vi "B_GetProperty.vi"(0 "reference in":refnum<class "Time.lvclass">, 5 "error in (no error)":errorcluster) -> (14 "reference out":refnum<class "Time.lvclass">, 15 "property":dbl, 19 "error out":errorcluster)   [LabVIEW 2018, in "Time.lvclass"]
uses:
  Time.lvclass
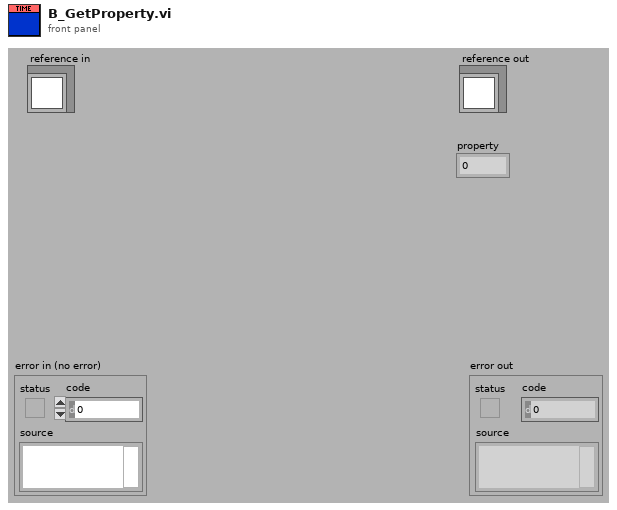
[diagram p1: front panel]
types:
  T1 = typedef "Time.lvclass/ObjectAttributes.ctl" = cluster{"Attribute1":dbl}
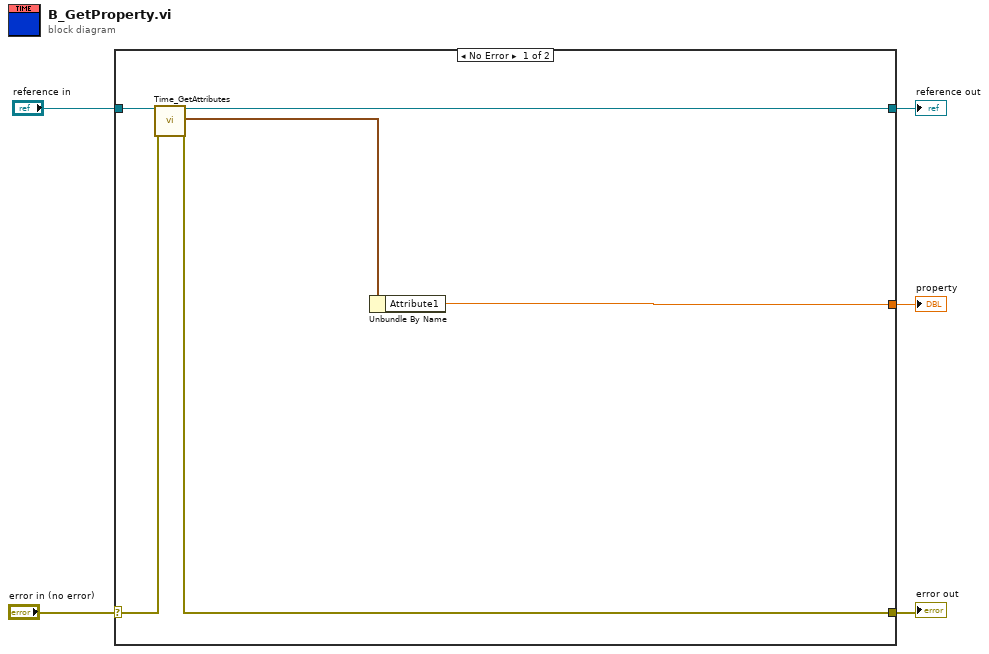
[diagram p0: block diagram]
diagram:
  n1 = case shown="No Error" "error in (no error)" {
    selector: "error in (no error)" -> [w11 w13]
    tunnel: [w9 w13] -> w4
    tunnel: [w7 w12] -> w2
    tunnel: "reference in" -> [w8 w12]
    tunnel: [w6 _] -> w1
    frame No Error {
      n2 = call "Time_GetAttributes.vi"("reference in"=w8, "error in (no error)"=w11) -> ("reference out"=w7:refnum<class "Time.lvclass">, "Attributes"=w10:T1, "error out"=w9:errorcluster)  [unwired: 14 in, 1 out]
      n3 = Unbundle By Name(w10) -> ("Attribute1"=w6:dbl)
    }
    frame Error {
    }
  }
  "error out" <- w4
  "reference out" <- w2
  "property" <- w1
